vi "Periodic Tasks.vi"() -> ()   [LabVIEW 2011]
doc: "This VI runs in parallel to other tasks. It can contain as many user-defined periodic loops as you need. These can carry out PID or other sorts of timed response."
uses:
  <vilib>/Rock Robotics/SystemInterfaces/Utilities/FPGA_UtilitiesLED State.ctl
  <vilib>/Rock Robotics/SystemInterfaces/Utilities/FPGA_UtilitiesLED Source.ctl
  <vilib>/Rock Robotics/WPI/Relay/WPI_RelayValue.ctl
  Robot Global Data.vi
panel:
  out "Ramp ACT Pot 2":dbl
  in  "Home Speed":dbl=1.0
  out "Auton Recording":bool
  in  "Turn on Record":bool
  in  "Auton Array":dbl[][](array[numeric])
  out "Right Rate":dbl
  out "Right Direction":bool
  out "Right Distance":dbl
  out "Shooter Encoder Distance":dbl
  out "Shooter Direction":bool
  out "Shooter Encoder Rate":dbl
  out "Left Rate":dbl
  out "Gyro Rate":dbl
  out "Gyro Angle":dbl
  out "Left Direction":bool
  out "Left Distance":dbl
  # "Auton Recording"
  # "Sensor Feedback"
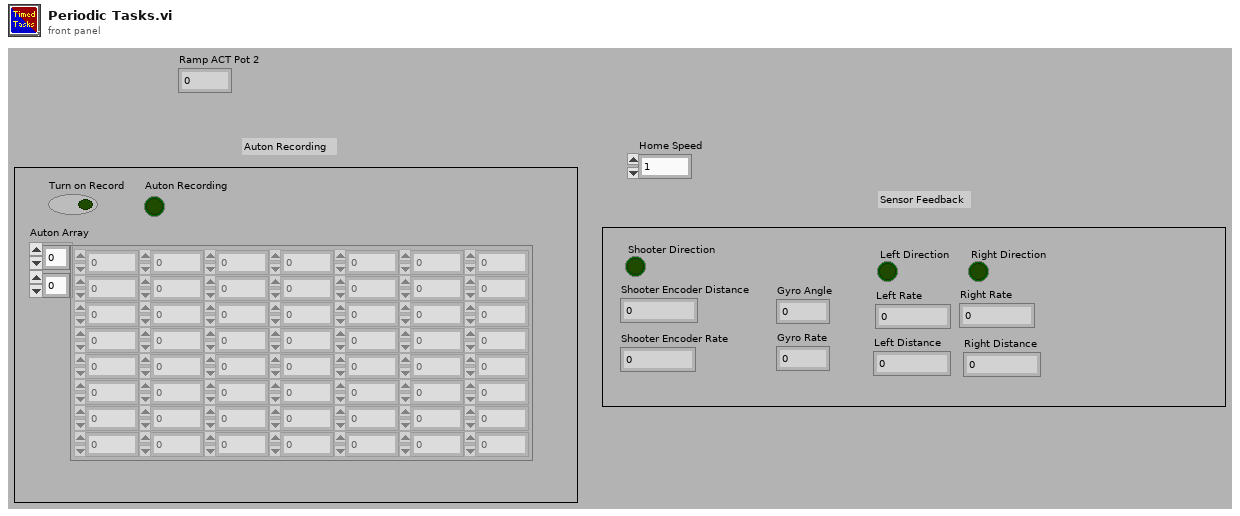
[diagram p1: front panel]
types:
  T1 = typedef "WPI_RelayValue.ctl" = enum16{"Off", "On", "Forward", "Reverse"}
  T2 = typedef "WPI_AnalogChannelDevRef.ctl" = cluster{"DevStatus":errorcluster, "Analog Module":T3, "Analog Channel":T4}
  T3 = typedef "FPGA_TypedefAnalogModule.ctl" = enum16{"Analog Module 1", "Analog Module 2"}
  T4 = typedef "FPGA_AIChannel.ctl" = enum8{"AI 1", "AI 2", "AI 3", "AI 4", "AI 5", "AI 6", "AI 7", "AI 8", "Invalid"}
  T5 = typedef "WPI_EncoderDevRef.ctl" = cluster{"DevStatus":errorcluster, "EncoderIndex":T6, "CounterIndex":T7, "DistancePerCount":dbl, "Decoding Type":T8}
  T6 = typedef "FPGA_EncoderIdx.ctl" = enum8{"Enc 0", "Enc 1", "Enc 2", "Enc 3", "Invalid"}
  T7 = typedef "FPGA_CounterCtrSystemIndex.ctl" = enum8{"Ctr 0", "Ctr 1", "Ctr 2", "Ctr 3", "Ctr 4", "Ctr 5", "Ctr 6", "Ctr 7", "Invalid"}
  T8 = typedef "WPI_EncoderType.ctl" = enum16{"1x", "2x", "4x"}
  T9 = typedef "WPI_GyroDevRef.ctl" = cluster{"DevStatus":errorcluster, "Analog Module":T3, "Analog Channel":T4, "Offset":dbl, "Gain (VoltsPerDegree/Second)":dbl}
  T10 = typedef "WPI_RelayDevRef.ctl" = cluster{"DevStatus":errorcluster, "Relay Channel":T11, "Digital Module":T12, "Relay Direction":T13}
  T11 = typedef "FPGA_DIORelayChannel.ctl" = enum8{"Relay 1", "Relay 2", "Relay 3", "Relay 4", "Relay 5", "Relay 6", "Relay 7", "Relay 8", "Invalid"}
  T12 = typedef "FPGA_TypedefDigitalModule.ctl" = enum16{"Digital Module 1", "Digital Module 2"}
  T13 = typedef "WPI_RelayDirection.ctl" = enum16{"Both directions", "Forward only", "Reverse only"}
  T14 = typedef "FPGA_UtilitiesLED State.ctl" = enum16{"Off", "On", "Toggle"}
  T15 = typedef "FPGA_UtilitiesLED Source.ctl" = enum16{"User LED", "FPGA LED"}
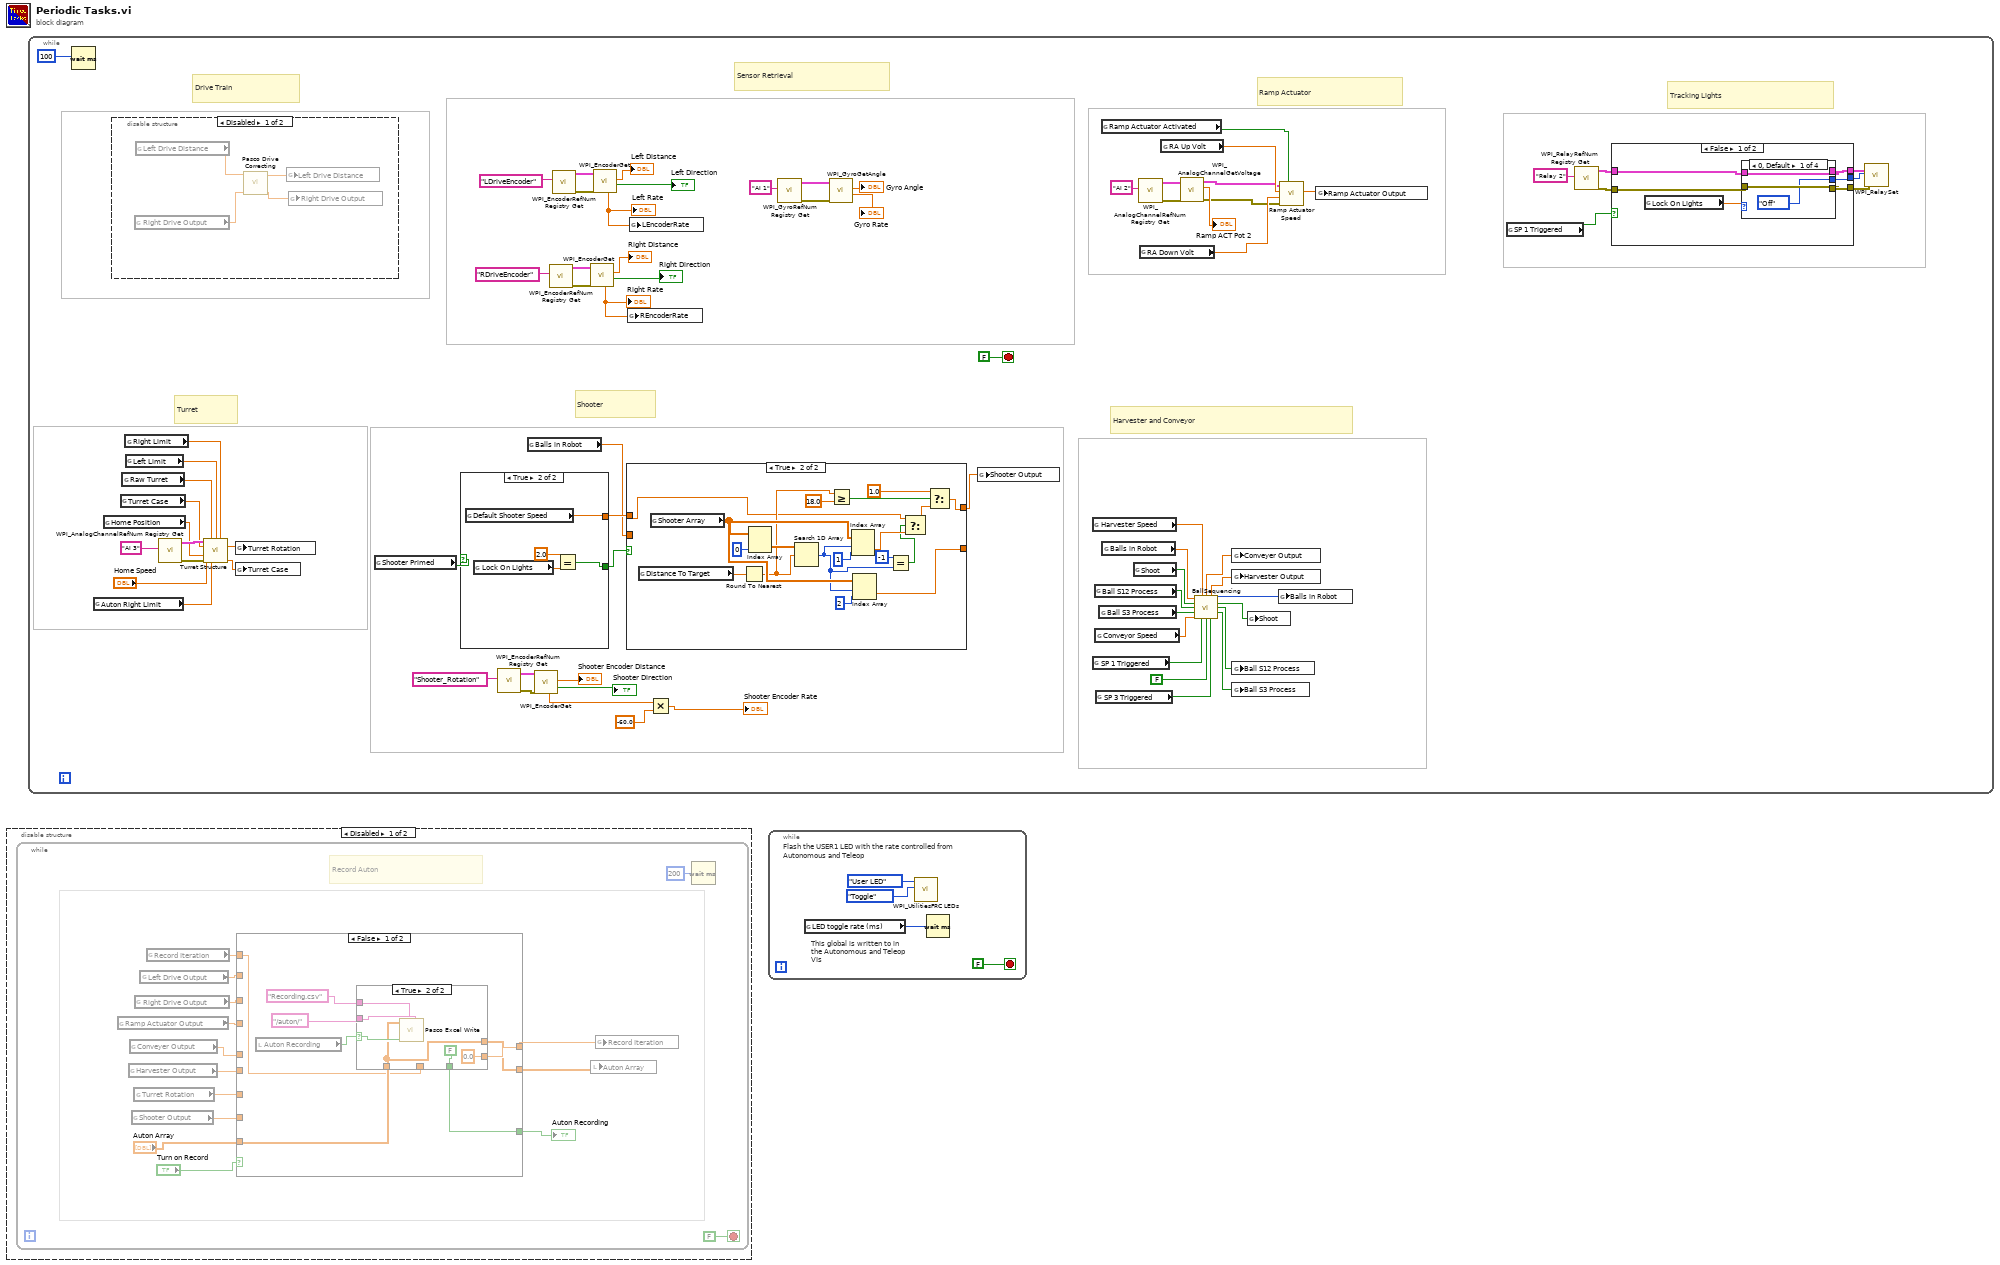
[diagram p0: block diagram]
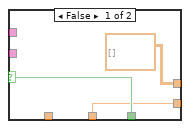
[diagram p2: hidden frame]
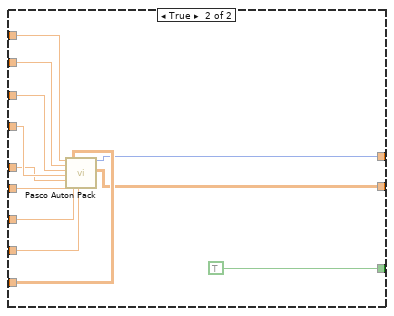
[diagram p3: hidden frame]
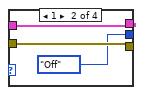
[diagram p5: hidden frame]
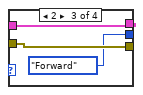
[diagram p6: hidden frame]
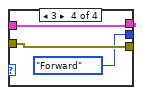
[diagram p7: hidden frame]
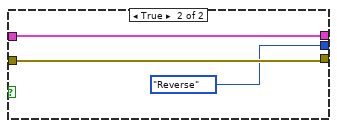
[diagram p8: hidden frame]
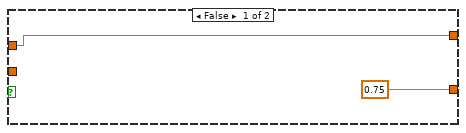
[diagram p9: hidden frame]
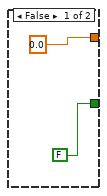
[diagram p10: hidden frame]
diagram:
  n1 = disable-structure shown="Disabled" {
    frame Disabled {
      n2 = while {
        stop <- FALSE stop-if-true
        # "Record Auton"
        n3 = global read "Robot Global Data.vi" "Ramp Actuator Output"() -> (w5:dbl)
        n4 = global read "Robot Global Data.vi" "Harvester Output"() -> (w7:dbl)
        n5 = global read "Robot Global Data.vi" "Conveyer Output"() -> (w6:dbl)
        n6 = global read "Robot Global Data.vi" "Shooter Output"() -> (w9:dbl)
        n7 = global read "Robot Global Data.vi" "Turret Rotation"() -> (w8:dbl)
        n8 = global read "Robot Global Data.vi" "Right Drive Output"() -> (w4:dbl)
        n9 = global read "Robot Global Data.vi" "Left Drive Output"() -> (w3:dbl)
        n10 = global read "Robot Global Data.vi" "Record Iteration"() -> (w2:dbl)
        n11 = case shown="False" "Turn on Record" {
          tunnel: w2 -> [w19 w44]
          tunnel: w3 -> [_ w43]
          tunnel: w4 -> [_ w42]
          tunnel: w5 -> [_ w41]
          tunnel: w6 -> [_ w40]
          tunnel: w7 -> [_ w39]
          tunnel: w8 -> [_ w38]
          tunnel: w9 -> [_ w37]
          tunnel: "Auton Array" -> [w20 w36]
          tunnel: [w16 w35] -> w12
          tunnel: [w17 w34] -> w13
          tunnel: [w18 TRUE] -> w14
          frame False {
            n12 = local read "Auton Recording"() -> (w21:bool)
            n13 = case shown="True" w21 {
              selector: w21 -> [w26 w31]
              tunnel: [w26 FALSE] -> w18
              tunnel: "/auton/" ("File Name") -> [_ w30]
              tunnel: "Recording.csv" ("Folder Location") -> [_ w29]
              tunnel: [w25 0.0 ("Record Iteration")] -> w17
              tunnel: w19 -> [w25 _]
              tunnel: w20 -> [_ w27]
              tunnel: [dbl[][] [] ("Auton Array") w27] -> w16
              frame False {
              }
              frame True {
                n14 = call "Pasco Excel Write.vi"("Folder Location"=w30, "File Name"=w29, "WriteToExcel"=w31, "2D data"=w27) -> ()  [unwired: 7 in, 1 out]
              }
            }
          }
          frame True {
            n15 = call "Pasco Auton Pack.vi"("Iterations"=w44, "Left Drive"=w43, "Right Drive"=w42, "RAMP ACT"=w41, "Conveyor"=w40, "Harvestor"=w39, "Auton Array"=w36, "Turret"=w38, "Shooter"=w37) -> ("Iteration Output"=w34:i32, "output array"=w35:dbl[][])  [unwired: 9 in]
          }
        }
        "Auton Recording" <- w14
        n16 = local write "Auton Array"(w12) -> ()
        n17 = global write "Robot Global Data.vi" "Record Iteration"(w13) -> ()
        n18 = Wait (ms)(milliseconds to wait=u32 200) -> ()  [unwired: 1 out]
      }
    }
    frame Enabled {
    }
  }
  n19 = while {
    stop <- FALSE stop-if-true
    # "Tracking Lights"
    # "Harvester and Conveyor"
    # "Shooter"
    # "Sensor Retrieval"
    # "Turret"
    # "Drive Train"
    # "Ramp Actuator"
    n20 = Wait (ms)(milliseconds to wait=u32 100) -> ()  [unwired: 1 out]
    n21 = global read "Robot Global Data.vi" "Auton Right Limit"() -> (w53:dbl)
    n22 = global read "Robot Global Data.vi" "Home Position"() -> (w114:dbl)
    n23 = disable-structure shown="Disabled" {
      frame Disabled {
        n24 = global read "Robot Global Data.vi" "Right Drive Output"() -> (w170:dbl)
        n25 = global read "Robot Global Data.vi" "Left Drive Distance"() -> (w171:dbl)
        n26 = call "Pasco Drive Correcting.vi"("RightDriveOutput"=w170, "LeftDriveOutput"=w171) -> ("RightDriveOutput"=w168:dbl, "LeftDriveOutput"=w169:dbl)  [unwired: 8 in]
        n27 = global write "Robot Global Data.vi" "Left Drive Distance"(w169) -> ()
        n28 = global write "Robot Global Data.vi" "Right Drive Output"(w168) -> ()
      }
      frame Enabled {
      }
    }
    n29 = global read "Robot Global Data.vi" "Turret Case"() -> (w115:dbl)
    n30 = global read "Robot Global Data.vi" "Raw Turret"() -> (w113:dbl)
    n31 = global read "Robot Global Data.vi" "Right Limit"() -> (w62:dbl)
    n32 = global read "Robot Global Data.vi" "Left Limit"() -> (w63:dbl)
    n33 = call <vilib>:"WPI_AnalogChannelRefNum Registry Get.vi"("refnum name"="AI 3") -> ("error out"=w116:errorcluster, "AIDeviceRef"=w117:T2)  [unwired: 9 in]
    n34 = call "Turret Structure.vi"("AIDeviceRef"=w117, "Raw Turret"=w113, "Left"=w63, "Right"=w62, "Turret Case"=w115, "Home Speed"="Home Speed", "Home postion"=w114, "error in (no error)"=w116, "Auton Right"=w53) -> ("Turret Output"=w112:dbl, "Turret Case Output"=w111:dbl)  [unwired: 5 in]
    n35 = global write "Robot Global Data.vi" "Turret Rotation"(w112) -> ()
    n36 = global write "Robot Global Data.vi" "Turret Case"(w111) -> ()
    n37 = global read "Robot Global Data.vi" "Shooter Primed"() -> (w98:bool)
    n38 = case shown="True" w98 {
      tunnel: [FALSE ("Shooter Primed") w165] -> w54
      tunnel: [0.0 w164] -> w96
      frame False {
      }
      frame True {
        n39 = global read "Robot Global Data.vi" "Default Shooter Speed"() -> (w164:dbl)
        n40 = global read "Robot Global Data.vi" "Lock On Lights"() -> (w167:dbl)
        n41 = Equal?(x=2.0, y=w167) -> (x = y?=w165:bool)
      }
    }
    n42 = call <vilib>:"WPI_EncoderRefNum Registry Get.vi"("refnum name"="Shooter_Rotation") -> ("error out"=w56:errorcluster, "EncoderDevRef"=w57:T5)  [unwired: 9 in]
    n43 = global read "Robot Global Data.vi" "Balls in Robot"() -> (w95:dbl)
    n44 = call <vilib>:"WPI_EncoderGet.vi"("error in (no error)"=w56, "EncoderDevRef"=w57) -> ("Direction"=→"Shooter Direction":bool, "Distance"=→"Shooter Encoder Distance":dbl, "Rate"=w52:dbl)  [unwired: 4 in, 3 out]
    n45 = call <vilib>:"WPI_EncoderRefNum Registry Get.vi"("refnum name"="RDriveEncoder") -> ("error out"=w78:errorcluster, "EncoderDevRef"=w77:T5)  [unwired: 9 in]
    n46 = call <vilib>:"WPI_EncoderRefNum Registry Get.vi"("refnum name"="LDriveEncoder") -> ("error out"=w84:errorcluster, "EncoderDevRef"=w83:T5)  [unwired: 9 in]
    n47 = call <vilib>:"WPI_EncoderGet.vi"("error in (no error)"=w78, "EncoderDevRef"=w77) -> ("Direction"=→"Right Direction":bool, "Distance"=→"Right Distance":dbl, "Rate"=w74:dbl)  [unwired: 4 in, 3 out]
    "Right Rate" <- w74
    n48 = call <vilib>:"WPI_EncoderGet.vi"("error in (no error)"=w84, "EncoderDevRef"=w83) -> ("Direction"=→"Left Direction":bool, "Distance"=→"Left Distance":dbl, "Rate"=w80:dbl)  [unwired: 4 in, 3 out]
    "Left Rate" <- w80
    n49 = case shown="True" w54 {
      tunnel: [w143 w152] -> w97
      tunnel: w96 -> [w143 w144]
      tunnel: w95 -> [_ _]
      tunnel: [0.75 w161] -> _
      frame False {
      }
      frame True {
        n50 = global read "Robot Global Data.vi" "Distance To Target"() -> (w158:dbl)
        n51 = global read "Robot Global Data.vi" "Shooter Array"() -> (w155:dbl[][])
        n52 = Round To Nearest(number=w158) -> (nearest integer value=w153:dbl)
        n53 = Index Array(array=w155, index (col)=0 ("disabled index (col)")) -> (element=w157:dbl[])  [unwired: 1 in]
        n54 = Search 1D Array(1D array=w157, element=w153) -> (index of element=w147:i32)  [unwired: 1 in]
        n55 = Greater Or Equal?(x=w153, y=18.0) -> (x >= y?=w151:bool)
        n56 = Index Array(array=w155, index (row)=w147, index (col)=1 ("disabled index (col)")) -> (element=w148:dbl)
        n57 = Index Array(array=w155, index (row)=w147, index (col)=2 ("disabled index (col)")) -> (element=w161:dbl)
        n58 = Equal?(x=-1, y=w147) -> (x = y?=w145:bool)
        n59 = Select(t=w144, s=w145, f=w148) -> (s? t:f=w149:dbl)
        n60 = Select(t=1.0, s=w151, f=w149) -> (s? t:f=w152:dbl)
      }
    }
    n61 = global write "Robot Global Data.vi" "REncoderRate"(w74) -> ()
    n62 = global write "Robot Global Data.vi" "LEncoderRate"(w80) -> ()
    n63 = Multiply(x=w52, y=-60.0) -> (x*y=→"Shooter Encoder Rate":dbl)
    n64 = call <vilib>:"WPI_GyroRefNum Registry Get.vi"("refnum name"="AI 1") -> ("error out"=w92:errorcluster, "GyroDevRef"=w93:T9)  [unwired: 9 in]
    n65 = call <vilib>:"WPI_GyroGetAngle.vi"("error in (no error)"=w92, "GyroDevRef"=w93) -> ("Angular Rate"=→"Gyro Rate":dbl, "Angle"=→"Gyro Angle":dbl)  [unwired: 6 in, 2 out]
    n66 = global write "Robot Global Data.vi" "Shooter Output"(w97) -> ()
    n67 = global read "Robot Global Data.vi" "Harvester Speed"() -> (w94:dbl)
    n68 = global read "Robot Global Data.vi" "SP 1 Triggered"() -> (w101:bool)
    n69 = global read "Robot Global Data.vi" "Ball S12 Process"() -> (w103:bool)
    n70 = global read "Robot Global Data.vi" "Conveyor Speed"() -> (w86:dbl)
    n71 = global read "Robot Global Data.vi" "SP 3 Triggered"() -> (w100:bool)
    n72 = global read "Robot Global Data.vi" "Ball S3 Process"() -> (w102:bool)
    n73 = global read "Robot Global Data.vi" "Ramp Actuator Activated"() -> (w69:bool)
    n74 = global read "Robot Global Data.vi" "Balls in Robot"() -> (w105:dbl)
    n75 = global read "Robot Global Data.vi" "Shoot"() -> (w104:bool)
    n76 = call <vilib>:"WPI_AnalogChannelRefNum Registry Get.vi"("refnum name"="AI 2") -> ("error out"=w67:errorcluster, "AIDeviceRef"=w68:T2)  [unwired: 9 in]
    n77 = global read "Robot Global Data.vi" "RA Down Volt"() -> (w72:dbl)
    n78 = global read "Robot Global Data.vi" "RA Up Volt"() -> (w71:dbl)
    n79 = call <vilib>:"WPI_AnalogChannelGetVoltage.vi"("error in (no error)"=w67, "AIDeviceRef"=w68) -> ("error out"=w64:errorcluster, "Voltage"=→"Ramp ACT Pot 2":dbl, "AIDeviceRef"=w65:T2)  [unwired: 7 in]
    n80 = call "BallSequencing.vi"("Balls In Robot"=w105, "Speed of Harvester"=w94, "Shoot"=w104, "Ball S12 Process"=w103, "Ball S3 Process"=w102, "Speed of Conveyor"=w86, "SP 1 Triggered"=w101, "SP 2 Triggered"=FALSE, "SP 3 Triggered"=w100) -> ("Conveyer Output"=w106:dbl, "Harvester Output"=w107:dbl, "Balls In Robot Output"=w88:i32, "Shoot Output"=w87:bool, "Ball S12 Process Output"=w109:bool, "Ball S3 Process Output"=w108:bool)  [unwired: 1 in]
    n81 = global write "Robot Global Data.vi" "Conveyer Output"(w106) -> ()
    n82 = global write "Robot Global Data.vi" "Harvester Output"(w107) -> ()
    n83 = global write "Robot Global Data.vi" "Ball S12 Process"(w109) -> ()
    n84 = global write "Robot Global Data.vi" "Ball S3 Process"(w108) -> ()
    n85 = global write "Robot Global Data.vi" "Shoot"(w87) -> ()
    n86 = global write "Robot Global Data.vi" "Balls in Robot"(w88) -> ()
    n87 = call "Ramp Actuator Speed.vi"("Up to Down"=w69, "error in (no error)"=w64, "RA Down Volt"=w72, "RA Up Volt"=w71, "AIDeviceRef"=w65) -> ("Ramp Actuator Ouput"=w70:dbl)  [unwired: 6 in]
    n88 = global write "Robot Global Data.vi" "Ramp Actuator Output"(w70) -> ()
    n89 = global read "Robot Global Data.vi" "SP 1 Triggered"() -> (w45:bool)
    n90 = call <vilib>:"WPI_RelayRefNum Registry Get.vi"("refnum name"="Relay 2") -> ("error out"=w47:errorcluster, "RelayDevRef"=w49:T10)  [unwired: 9 in]
    n91 = case shown="False" w45 {
      tunnel: [w126 w141] -> w50
      tunnel: w49 -> [w125 w141]
      tunnel: [w124 w140] -> w48
      tunnel: w47 -> [w123 w140]
      tunnel: [w122 WPI_RelayValue."Reverse" ("RelayValue")] -> w46
      frame False {
        n92 = global read "Robot Global Data.vi" "Lock On Lights"() -> (w121:dbl)
        n93 = case shown="0, Default" w121 {
          tunnel: [w129 w132 w135 w138] -> w126
          tunnel: w125 -> [w129 w132 w135 w138]
          tunnel: [w128 w131 w134 w137] -> w124
          tunnel: w123 -> [w128 w131 w134 w137]
          tunnel: [WPI_RelayValue."Off" ("RelayValue") WPI_RelayValue."Off" ("RelayValue") WPI_RelayValue."Forward" ("RelayValue") WPI_RelayValue."Forward" ("RelayValue")] -> w122
          frame 0, Default {
          }
          frame 1 {
          }
          frame 2 {
          }
          frame 3 {
          }
        }
      }
      frame True {
      }
    }
    n94 = call <vilib>:"WPI_RelaySet.vi"("error in (no error)"=w48, "RelayValue"=w46, "RelayDevRef"=w50) -> ()  [unwired: 7 in, 2 out]
  }
  n95 = while {
    stop <- FALSE stop-if-true
    # "This global is written to in the Autonomous and Teleop VIs"
    # "Flash the USER1 LED with the rate controlled from Autonomous and Teleop"
    n96 = global read "Robot Global Data.vi" "LED toggle rate (ms)"() -> (w172:u32)
    n97 = call <vilib>:"WPI_UtilitiesFRC LEDs.vi"("State"=FPGA_UtilitiesLED_State."Toggle", "LED Type"=FPGA_UtilitiesLED_Source."User LED") -> ()  [unwired: 1 in, 9 out]
    n98 = Wait (ms)(milliseconds to wait=w172) -> ()  [unwired: 1 out]
  }
